vi "rad_ViewInstalledSoftware.vi"(11 "Installed Software":string) -> ()   [LabVIEW 2020]
panel:
  in  "Close":bool
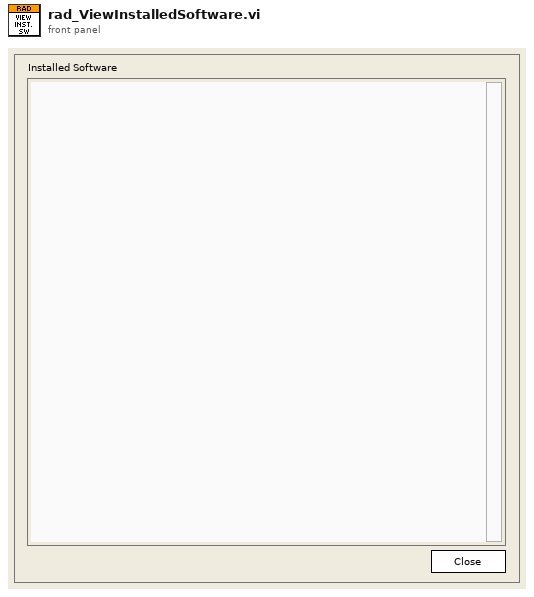
[diagram p1: front panel]
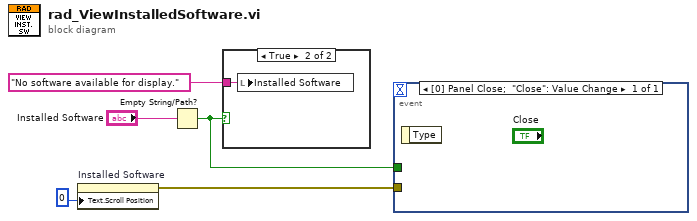
[diagram p0: block diagram]
diagram:
  n1 = property on="Installed Software" class="Str"("Text.Scroll Position"=u32 0) -> (error out=w1:errorcluster)  [unwired: 2 in, 1 out]
  n2 = Empty String/Path?(string/path="Installed Software") -> (empty?=w2:bool)
  n3 = case shown="True" w2 {
    tunnel: "No software available for display." ("Installed Software") -> [_ w6]
    frame False {
    }
    frame True {
      n4 = local write "Installed Software"(w6) -> ()
    }
  }
  n5 = event shown="[0] Panel Close;  \"Close\": Value Change" {
    selector: _ -> [_]
    dyn-events: _ -> [_]
    timeout: _ -> [_]
    tunnel: w2 -> [_]
    tunnel: w1 -> [_]
    event Panel Close; "Close": Value Change {
      n6 = event-data() -> ()  [unwired: 1 in, 1 out]
    }
  }
